vi "多参数全局变量.vi"() -> ()   [LabVIEW 2016, in "斯坦道多参数.lvlib"]
uses:
  <vilib>/Plasmionique/MB Master/MB_Master/MB_Master.lvclass
panel:
  out "配置文件 path":path
  out "ping":bool
  out "副屏状态":u16(ring) items=["空闲", "水样测试", "标样核查", "停止"]
  out "主屏状态":u16(ring) items=["空闲", "水样测试", "标样核查", "停止"]
  in  "副屏IP":cluster{"address":string, "port (502)":u16}={"address"="192.168.1.101", "port (502)"=100}
  out "主副屏同步启动":u16(ring) items=["空闲", "水样测试", "标样核查", "停止"]
  in  "主屏IP":cluster{"address":string, "port (502)":u16}={"address"="192.168.1.100", "port (502)"=100}
  out "蓝绿藻通讯状态":bool
  out "藻密度通讯状态":bool
  out "叶绿素a通讯状态":bool
  out "浊度通讯状态":bool
  out "spcond通讯状态":bool
  out "DO通讯状态":bool
  out "ph通讯状态":bool
  in  "校准VI引用句柄":T1
  in  "MB session in":refnum<class "MB_Master.lvclass">
  in  "运行模式":enum16{"维护模式", "常规模式", "应急模式", "质控模式"}(ring)=enum."常规模式"
  in  "多参数编号":string
  out "藻密度显示":cluster{"温度测量值":sgl, "测量值":sgl, "温度偏移修正值":sgl}
  out "蓝绿藻显示":cluster{"温度测量值":sgl, "测量值":sgl, "温度偏移修正值":sgl}
  out "cond显示":cluster{"温度测量值":sgl, "测量值":sgl, "温度偏移修正值":sgl}
  out "盐度显示":cluster{"温度测量值":sgl, "测量值":sgl, "温度偏移修正值":sgl}
  out "spcond显示":cluster{"温度测量值":sgl, "测量值":sgl, "温度偏移修正值":sgl}
  out "ph显示":cluster{"温度测量值":sgl, "测量值":sgl, "温度偏移修正值":sgl}
  out "水温显示":cluster{"CH":u16, "监测值":dbl, "温度偏移修正值":sgl}={"CH"=1, "监测值"=0.0, "温度偏移修正值"=0.0} {"CH" items=["pH", "Cond", "DO", "Turb"]}
  out "浊度显示":cluster{"温度测量值":sgl, "测量值":sgl, "温度偏移修正值":sgl}
  out "DO显示":T2
  out "叶绿素a显示":cluster{"温度测量值":sgl, "测量值":sgl, "温度偏移修正值":sgl}
  out "多参数运行状态":u16(ring) items=["空闲", "水样测试", "标样核查"]
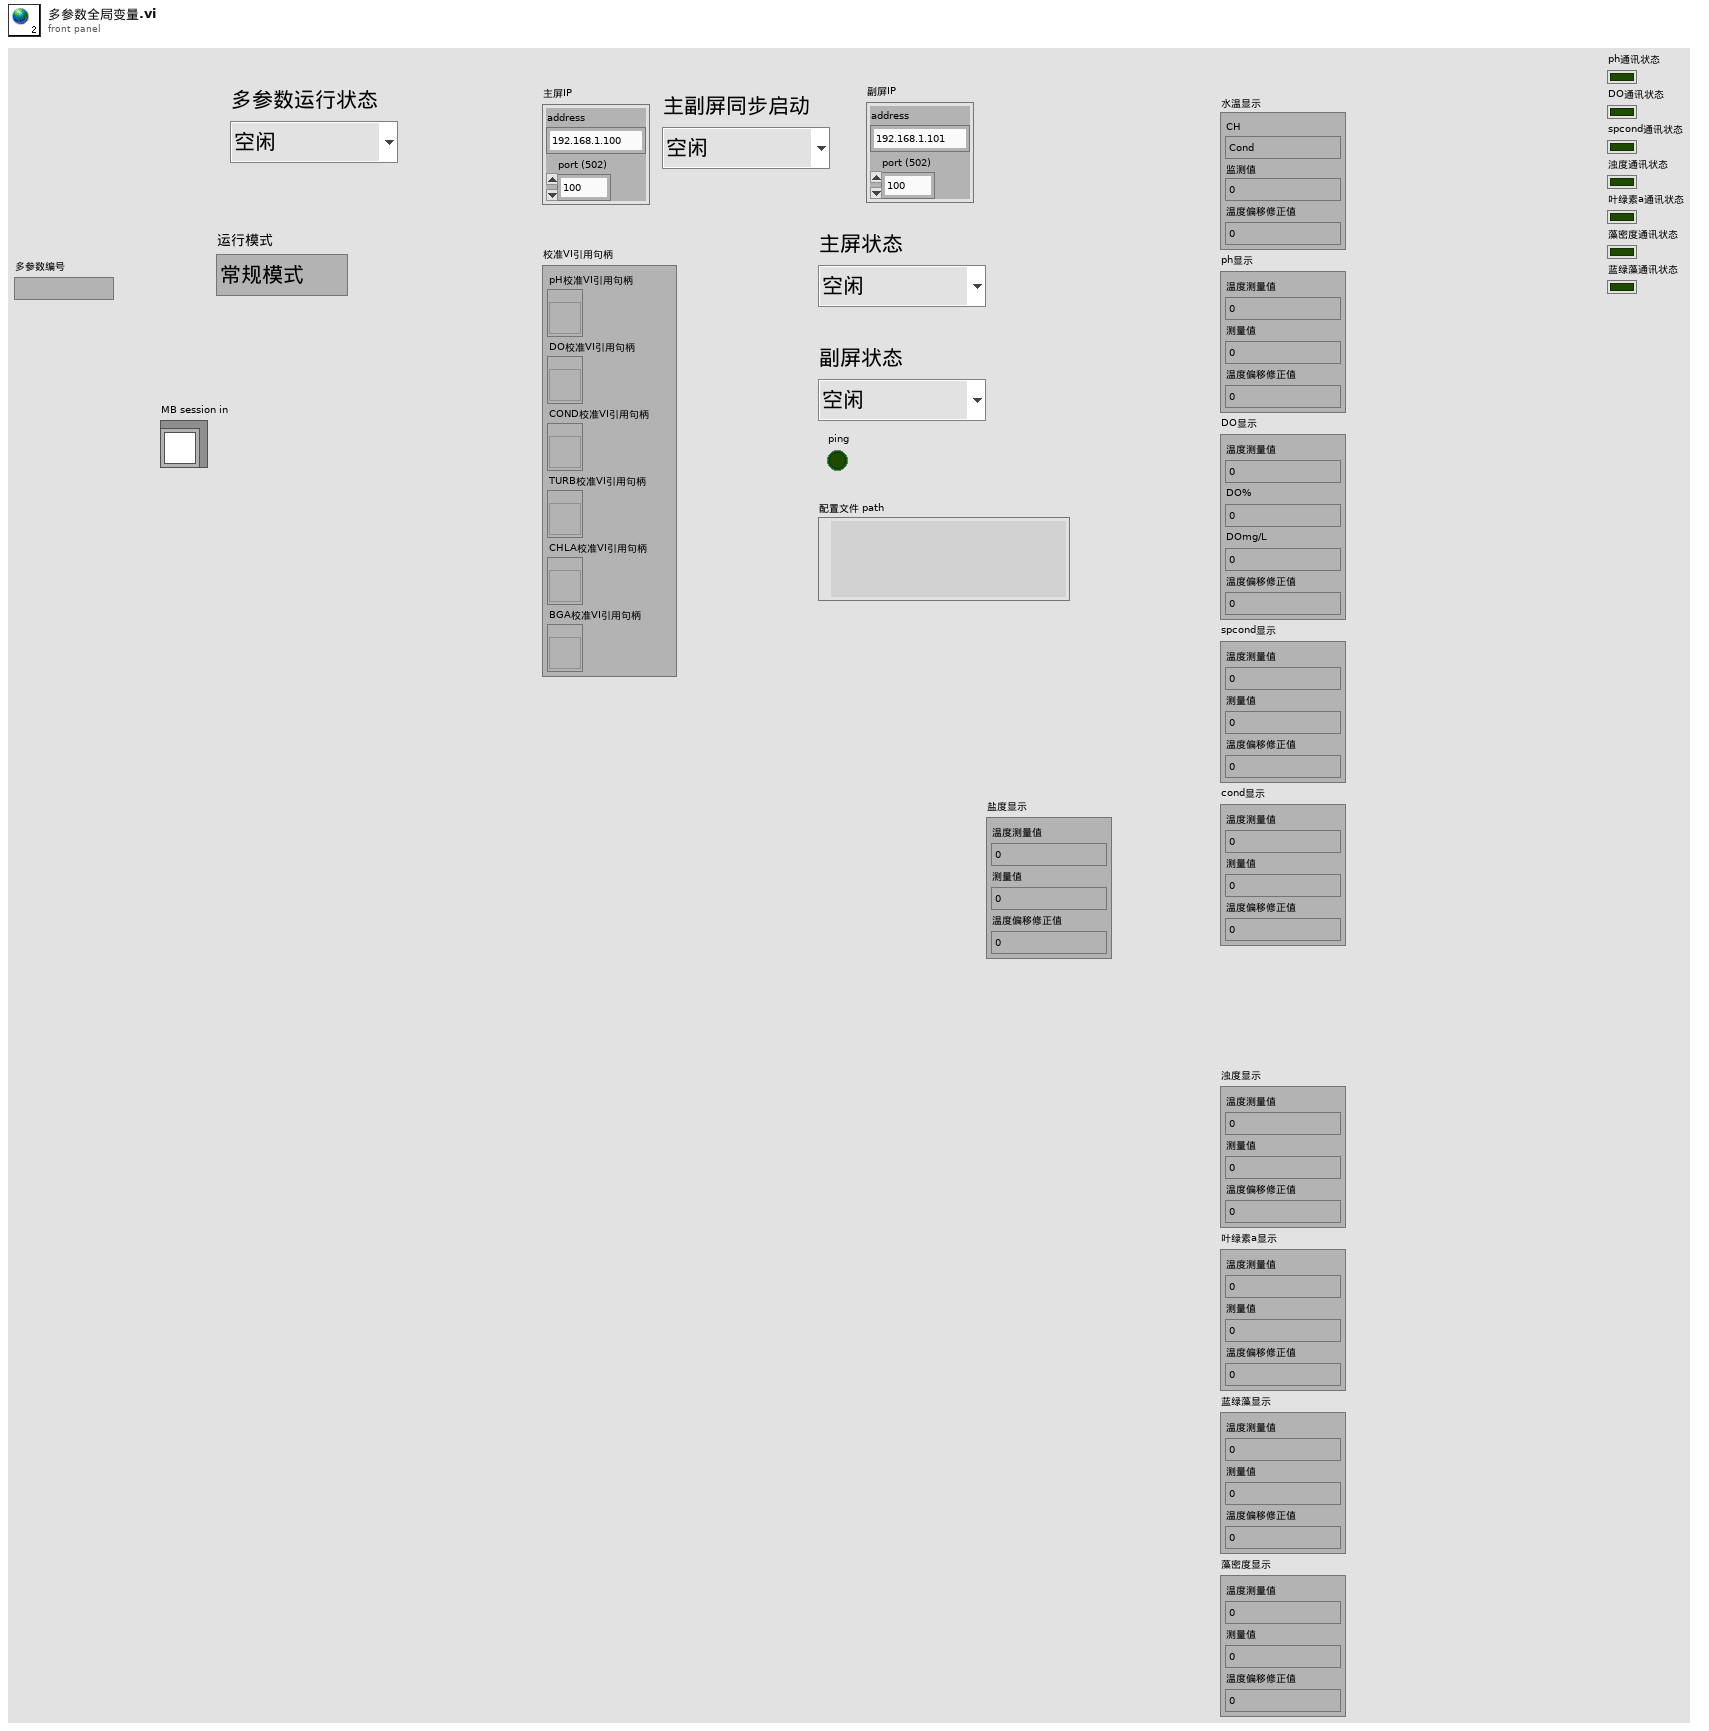
[diagram p1: front panel]
types:
  T1 = cluster{"pH校准VI引用句柄":refnum<vi>, "DO校准VI引用句柄":refnum<vi>, "COND校准VI引用句柄":refnum<vi>, "TURB校准VI引用句柄":refnum<vi>, "CHLA校准VI引用句柄":refnum<vi>, "BGA校准VI引用句柄":refnum<vi>}
  T2 = cluster{"温度测量值":sgl, "DO%":sgl, "DOmg/L":sgl, "温度偏移修正值":sgl}
diagram:
